vi "test_Create Global MetaData Channel_array format.vi"(8 "error in (no error)":errorcluster, 11 "TestCase in":refnum<class "Instrument Addon Scripting API Channels Unit Tests.lvclass">) -> (0 "error out":errorcluster, 3 "TestCase out":refnum<class "Instrument Addon Scripting API Channels Unit Tests.lvclass">)   [LabVIEW 2019, in "Instrument Addon Scripting API Channels Unit Tests.lvclass"]
uses:
  Instrument Addon Scripting API Channels Unit Tests.lvclass
  <vilib>/addons/_JKI Toolkits/VI Tester/TestCase.llb/TestCase.lvclass
  <vilib>/NI VeriStand/Custom Device Tools/Custom Device Utility Library/Custom Device Utility Library.lvlib
  Addon/Addon Shared/SubVIs/Constants.vi
  Addon/Addon Shared/Instrument Addon Shared.lvlib
  Addon/Addon Shared/Types/FG Control.ctl
  APIs/Scripting API/Instrument Addon Scripting API.lvlib
  APIs/Scripting API/TypeDefs/Array Element.ctl
  APIs/Scripting API/TypeDefs/Array Format Settings.ctl
  APIs/Scripting API/Channels/Create Global MetaData Channel - Array - Format.vi
  <vilib>/NI VeriStand/Custom Device Tools/Custom Device Utility Library/NI VeriStand - Search for Item by Name.vi
  <vilib>/NI VeriStand/Custom Device Tools/Custom Device Utility Library/NI VeriStand - Search for Item by GUID.vi
  C:/Program Files (x86)/National Instruments/LabVIEW 2019/vi.lib/addons/_JKI Toolkits/VI Tester/TestCase.llb/TestCase.lvclass
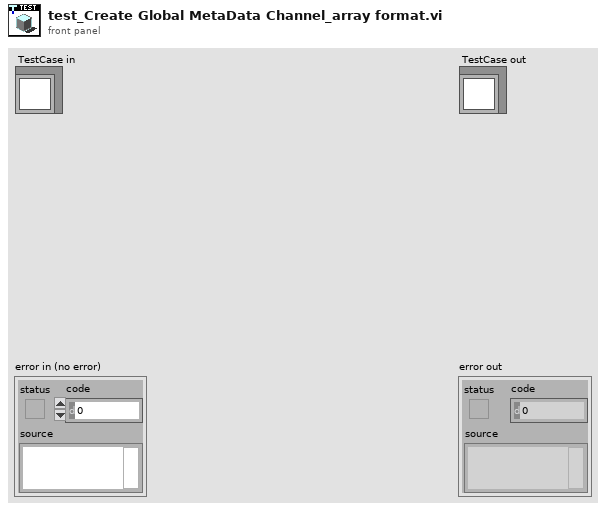
[diagram p1: front panel]
types:
  T1 = typedef "Instrument Addon Shared.lvlib/FG Control.ctl" = enum16{"Get", "Set"}
  T2 = typedef "Instrument Addon Scripting API.lvlib/Array Format Settings.ctl" = cluster{"Elements":T3[], "Format String":string, "Delimiter":string}
  T3 = typedef "Instrument Addon Scripting API.lvlib/Array Element.ctl" = cluster{"Name":string, "Default Value":dbl, "Units":string}
  T4 = typedef "Custom Device API.lvlib/Custom Device Item Ref.ctl" = u64
  T5 = typedef "Instrument Addon Shared.lvlib/MetaData Parameters.ctl" = cluster{"Data Type":T6, "Channel Type":T7, "List":string[], "Format String":string, "Type":T8, "Delimiter":string, "Endian":T9}
  T6 = typedef "Instrument Addon Shared.lvlib/Protocol Data Type.ctl" = enum16{"Single Channel", "Array"}
  T7 = typedef "Instrument Addon Shared.lvlib/Metadata Channel Type.ctl" = enum16{"Enumerated List", "Format", "Type Cast"}
  T8 = typedef "Instrument Addon Shared.lvlib/Type Cast Type.ctl" = enum16{"DBL", "SGL", "U64", "U32", "U16", "U8", "I64", "I32", "I16", "I8"}
  T9 = typedef "Instrument Addon Shared.lvlib/Endian.ctl" = enum16{"Native", "Little", "Big"}
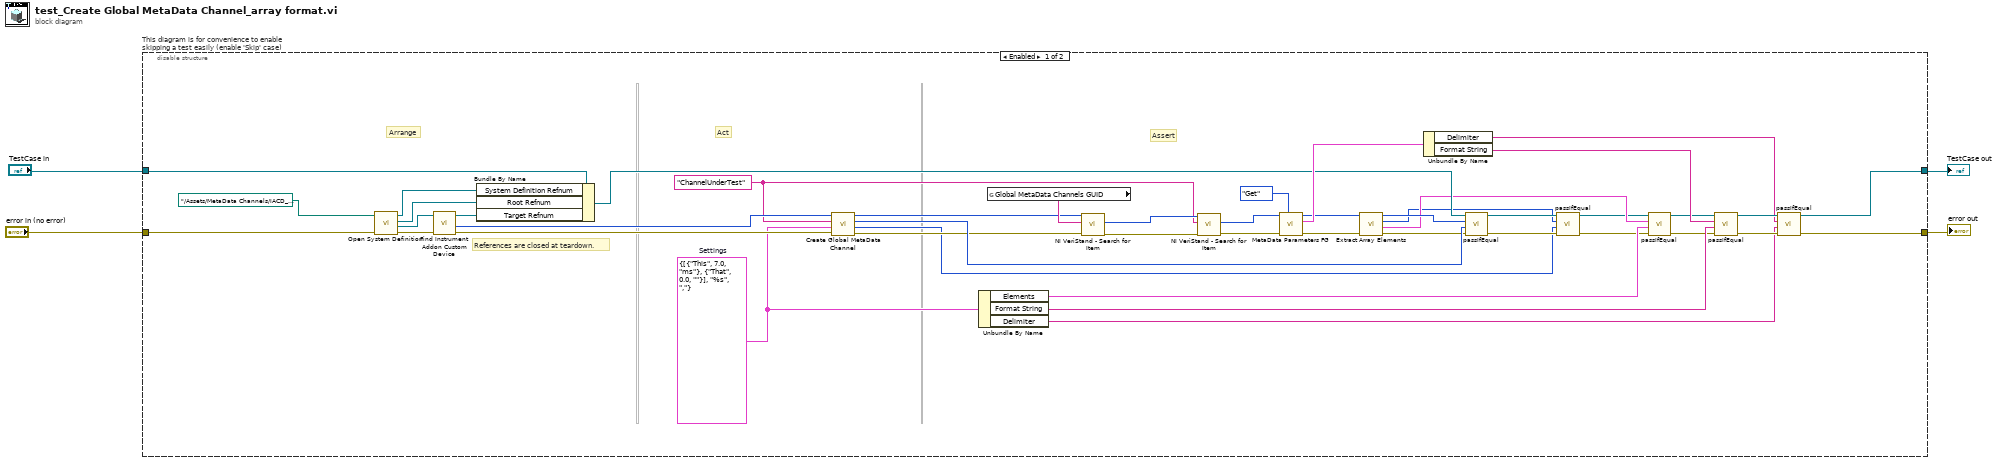
[diagram p0: block diagram]
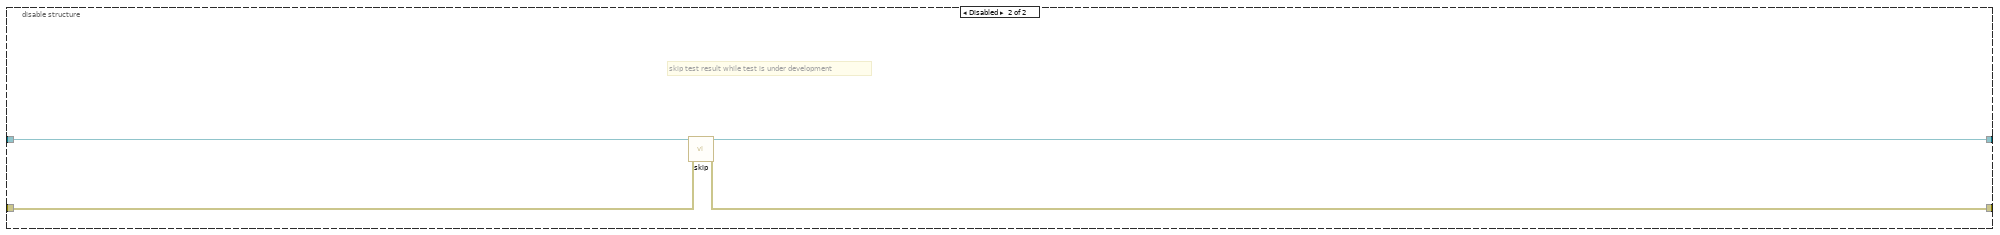
[diagram p2: hidden frame]
diagram:
  n1 = disable-structure "This diagram is for convenience to enable skipping a test easily (enable 'Skip' case)" shown="Enabled" {
    disable-tunnel: "TestCase in" -> [w31 w53]
    disable-tunnel: [w22 w51] -> w1
    disable-tunnel: [w21 w52] -> w3
    disable-tunnel: "error in (no error)" -> [w49 w50]
    frame Enabled {
      w13 = T2 {"Elements"=[{"Name"="This", "Default Value"=7.0, "Units"="ms"}, {"Name"="That", "Default Value"=0.0, "Units"=""}], "Format String"="%s", "Delimiter"=","}  # Settings
      w29 = "ChannelUnderTest" ("Name")
      # "References are closed at teardown."
      # "Assert"
      # "Act"
      # "Arrange"
      n2 = call "Open System Definition.vi"("error in (no error)"=w49, "System Definition File"=path "../Assets/MetaData Channels/IACD_channels.nivssdf") -> ("error out"=w47:errorcluster, "Target Refnum"=w48:refnum<k24>, "Root Refnum"=w34:refnum<k24>, "System Definition Refnum"=w33:refnum<k24>)  [unwired: 6 in]
      n3 = call "Find Instrument Addon Custom Device.vi"("error in"=w47, "target in"=w48) -> ("error out"=w28:errorcluster, "NodeID"=w30:u64, "target out"=w35:refnum<k24>)  [unwired: 7 in]
      n4 = Bundle By Name(cluster=w31, "System Definition Refnum"=w33, "Root Refnum"=w34, "Target Refnum"=w35) -> (w32:refnum<class "Instrument Addon Scripting API Channels Unit Tests.lvclass">)
      n5 = call-poly "Create Global MetaData Channel.vi"("error in (no error)"=w28, "settings"=w13, "channel name"=w29, "instrument addon refnum in"=w30) -> ("error out"=w25:errorcluster, "channel refnums"=w6:T4[], "array refnum"=w26:T4, "instrument addon refnum out"=w27:T4)  [unwired: 4 in]
      n6 = Unbundle By Name(w13) -> ("Elements"=w18:T3[], "Format String"=w36:string, "Delimiter"=w24:string)
      n7 = global read "Constants.vi" "Global MetaData Channels GUID"() -> (w46:string)
      n8 = call-poly <vilib>:"NI VeriStand - Search for Item.vi"("error in"=w25, "Item GUID"=w46, "Section Ref in"=w27) -> ("error out"=w44:errorcluster, "Item Ref"=w45:T4)  [unwired: 5 in, 2 out]
      n9 = call-poly <vilib>:"NI VeriStand - Search for Item.vi"("error in"=w44, "Item Name"=w29, "Section Ref in"=w45) -> ("error out"=w43:errorcluster, "Item Ref"=w42:T4)  [unwired: 5 in, 2 out]
      n10 = call "MetaData Parameters FG.vi"("Action"=FG_Control."Get", "error in (no error)"=w43, "Item Ref in"=w42) -> ("error out"=w17:errorcluster, "MetaData Parameters"=w40:T5, "Item Ref out"=w16:T4)  [unwired: 6 in]
      n11 = call "Extract Array Elements.vi"("error in (no error)"=w17, "array reference in"=w16) -> ("error out"=w15:errorcluster, "elements"=w12:T3[], "channel refnums"=w7:T4[], "array reference out"=w14:T4)  [unwired: 6 in]
      n12 = Unbundle By Name(w40) -> ("Delimiter"=w23:string, "Format String"=w37:string)
      n13 = call-dynamic "passIfEqual.vi"("error in (no error)"=w15, "y"=w26, "x"=w14, "TestCase in"=w32) -> ("error out"=w9:errorcluster, "TestCase out"=w11:refnum<class "Instrument Addon Scripting API Channels Unit Tests.lvclass">)  [unwired: 6 in]
      n14 = call-dynamic "passIfEqual.vi"("error in (no error)"=w9, "y"=w6, "x"=w7, "TestCase in"=w11) -> ("error out"=w8:errorcluster, "TestCase out"=w10:refnum<class "Instrument Addon Scripting API Channels Unit Tests.lvclass">)  [unwired: 6 in]
      n15 = call-dynamic "passIfEqual.vi"("error in (no error)"=w8, "y"=w18, "x"=w12, "TestCase in"=w10) -> ("error out"=w19:errorcluster, "TestCase out"=w20:refnum<class "Instrument Addon Scripting API Channels Unit Tests.lvclass">)  [unwired: 6 in]
      n16 = call-dynamic "passIfEqual.vi"("error in (no error)"=w19, "y"=w36, "x"=w37, "TestCase in"=w20) -> ("error out"=w39:errorcluster, "TestCase out"=w38:refnum<class "Instrument Addon Scripting API Channels Unit Tests.lvclass">)  [unwired: 6 in]
      n17 = call-dynamic "passIfEqual.vi"("error in (no error)"=w39, "y"=w24, "x"=w23, "TestCase in"=w38) -> ("error out"=w21:errorcluster, "TestCase out"=w22:refnum<class "Instrument Addon Scripting API Channels Unit Tests.lvclass">)  [unwired: 6 in]
    }
    frame Disabled {
      # "skip test result while test is under development"
      n18 = call <vilib>:"skip.vi"("error in (no error)"=w50, "TestCase in"=w53) -> ("error out"=w52:errorcluster, "TestCase out"=w51:refnum<class "Instrument Addon Scripting API Channels Unit Tests.lvclass">)  [unwired: 8 in]
    }
  }
  "error out" <- w3
  "TestCase out" <- w1
